vi "Status_ExcelDecode.vi"(8 "error in (no error)":errorcluster, 11 "2D Data":string[][](array[string])) -> (0 "error out":errorcluster)   [LabVIEW 2015]
uses:
  Control 1.ctl
  g_variable/g_Excel Attributes.vi
  MemberAttendance/MemberAttendance.lvclass
panel:
  in  "MemberAttendance":refnum<class "MemberAttendance.lvclass">
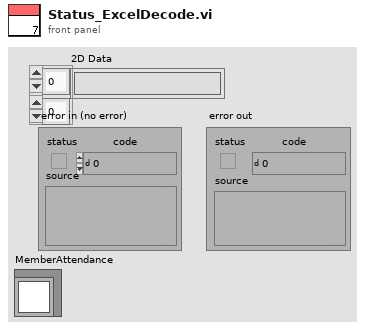
[diagram p1: front panel]
types:
  T1 = typedef "Control 1.ctl" = enum16{"姓名", "部门", "周次", "数据"}
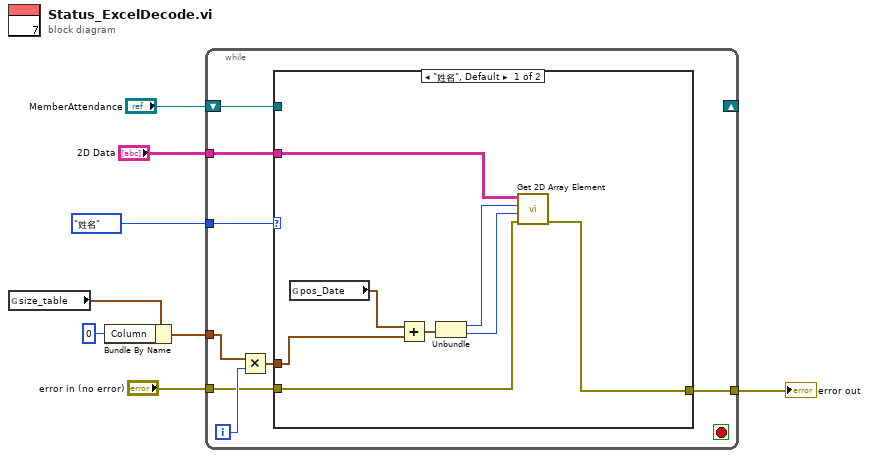
[diagram p0: block diagram]
diagram:
  n1 = global read "g_Excel Attributes.vi" "size_table"() -> (w6:cluster{"Column":i32, "Row":i32})
  n2 = Bundle By Name(cluster=w6, "Column"=0) -> (w4:cluster{"Column":i32, "Row":i32})
  n3 = while {
    tunnel: Control_1."姓名" -> [w16]
    tunnel: "2D Data" -> [w15]
    tunnel: w4 -> [w14]
    tunnel: "error in (no error)" -> [w11]
    tunnel: [w10] -> w2
    shift-right: _ -> [_]
    shift-left: "MemberAttendance" -> [w9]
    i -> [w13]
    stop <- _ stop-if-true
    n4 = Multiply(x=w14, y=w13) -> (x*y=w12:cluster{"Column":i32, "Row":i32})
    n5 = case shown="\"姓名\", Default" w16 {
      tunnel: w15 -> [w21 _]
      tunnel: w12 -> [w23 _]
      tunnel: w11 -> [w18 _]
      tunnel: [w17 _] -> w10
      tunnel: w9 -> [_ _]
      frame "姓名", Default {
        n6 = global read "g_Excel Attributes.vi" "pos_Date"() -> (w24:cluster{"x":i32, "y":i32})
        n7 = Add(x=w24, y=w23) -> (x+y=w22:cluster{i32, i32})
        n8 = Unbundle(w22) -> (w20:i32, w19:i32)
        n9 = call "Get 2D Array Element.vi"("error in (no error)"=w18, "Col"=w19, "Row"=w20, "Array"=w21) -> ("error out"=w17:errorcluster)  [unwired: 5 in, 2 out]
      }
      frame "部门" {
      }
    }
  }
  "error out" <- w2
